vi "Save Metadata.vi"(8 "error in (no error)":errorcluster, 10 "Metadata.lvclass":refnum<class "Metadata.lvclass">, 11 "File in":refnum<class "File.lvclass">) -> (0 "error out":errorcluster, 1 "channel name out":string, 2 "group name out":string, 3 "File out":refnum<class "File.lvclass">)   [LabVIEW 2024, in "File.lvclass"]
uses:
  File.lvclass
  File.lvclass/File.ctl
  Read tdms stream.vi
  Write tdms stream.vi
  Metadata/Metadata.lvclass
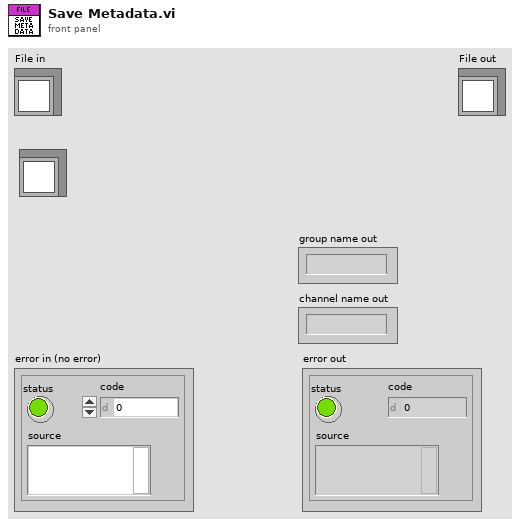
[diagram p1: front panel]
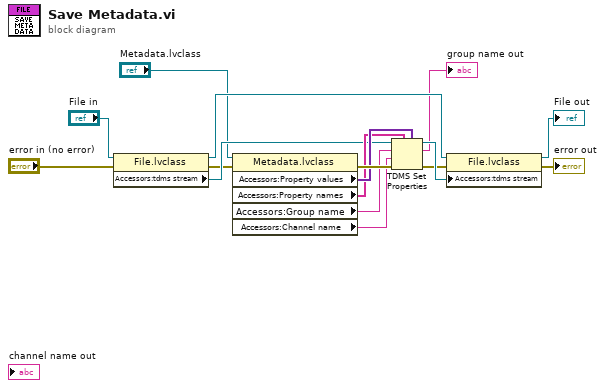
[diagram p0: block diagram]
diagram:
  n1 = property class="File.lvclass"(reference="File in", error in="error in (no error)") -> (reference out=w14:refnum<class "File.lvclass">, error out=w4:errorcluster, "Accessors:tdms stream"=w6:refnum<k34>)
  n2 = property class="Metadata.lvclass"(reference="Metadata.lvclass", error in=w4) -> (error out=w11:errorcluster, "Accessors:Property values"=w10:variant[], "Accessors:Property names"=w9:string[], "Accessors:Group name"=w8:string, "Accessors:Channel name"=w7:string)  [unwired: 1 out]
  n3 = TDMS Set Properties(5:w10, 7:w9, 8:w11, 9:w7, 10:w8, 11:w6) -> (0:w1:errorcluster, 2:→"group name out":string, 3:w5:refnum<k34>)  [unwired: 1 out]
  n4 = property class="File.lvclass"(reference=w14, error in=w1, "Accessors:tdms stream"=w5) -> (reference out=→"File out":refnum<class "File.lvclass">, error out=→"error out":errorcluster)
